vi "Protocol.Initialize.vi"(8 "error in (no error)":errorcluster, 10 "Parameters in":T21={"Name"="", "XNET.Settings"={"Database"="", "Cluster"="", "Port"="", "Baud rate [Bd]"=0, "Termination"=0, "Incoming Decimation"=0, "Outgoing Decimation"=1}, "Monitor.Network"={"Address"=0, "Name"=0, "Include DA"=FALSE}, "Data"=[], "DTCs"=[], "Sim.Nodes.LUT"=variant, "Data.LUT"=variant, "PCL"=0} {"Monitor.Network"."Name" format="%.0x"; "DTCs"."Data"."DM1.Ref"."Data Reference" format="%.0x"; "DTCs"."Data"."DM1.Enable.Ref"."Data Reference" format="%.0x"; "DTCs"."Data"."DM2.Ref"."Data Reference" format="%.0x"; "DTCs"."Data"."DM2.Enable.Ref"."Data Reference" format="%.0x"; "Data"."Trigger.Refs"."Data Reference" format="%.0x"; "Data"."Disable.Refs"."Data Reference" format="%.0x"; "Data"."Timing.Refs"."Data Reference" format="%.0x"; "Data"."Network"."Name" format="%.0x"; "Data"."Incoming.Refs"."Data Reference" format="%.0x"; "Data"."Outgoing.Refs"."Data Reference" format="%.0x"; "XNET.Settings"."Termination" items=["Off", "On"]}, 11 "Process":refnum<class "Process.lvclass">) -> (0 "error out":errorcluster, 2 "Notification":bool, 3 "Protocol State Variables":T1 {"Stream Refs"."Port Settings"."FD ISO Mode" items=["ISO", "Non ISO", "ISO Legacy"]; "Stream Refs"."Port Settings"."Termination" items=["Off", "On"]; "Stream Refs"."Port Settings"."Mode" items=["CAN 2.0", "CAN FD", "CAN FD+BRS"]})   [LabVIEW 2019, in "J1939 Addon Engine.lvlib"]
uses:
  J1939 Addon Engine.lvlib
  Support Libraries/J1939 Utilities/Types/CAN Outgoing Message Cluster.ctl
  Support Libraries/J1939 Utilities/J1939 Utilities.lvlib
  Types/Protocol.Refs.ctl
  Types/Protocol.Configuration.ctl
  Types/Protocol.XNET Settings.ctl
  Types/Protocol.Address Table Reference.ctl
  Types/Protocol.RQST Lookup Table Reference.ctl
  <vilib>/NI/NI VeriStand Addon Network Comm/Engine/VeriStand Comm.lvclass
  <vilib>/NI/NIVS Inline Async API/_VS Inline Async API/Process/Process.lvclass
  <vilib>/NI/NIVS Inline Async API/_Data Access Engine/Access Type Classes/Write/Write.lvclass
  <vilib>/NI/NIVS Inline Async API/_Data Access Engine/Data Access Engine/Types/Write.DVR.ctl
  <vilib>/NI/NIVS Inline Async API/_Data Access Engine/Data Access Engine/Data Access Engine.lvclass
  <vilib>/NI/NIVS Inline Async API/_Data Access Engine/Access Type Classes/Read/Read.lvclass
  <vilib>/NI/NIVS Inline Async API/_Data Access Engine/Data Access Engine/Types/Read.DVR.ctl
  Addon Shared/SubVIs/Constants.vi
  Addon Shared/J1939 Addon Shared.lvlib
  SubModules/Frame-Protection-Support/Source/Engine/Types/RT Frame Settings.ctl
  SubModules/Frame-Protection-Support/Source/Engine/Protection and Counter Support Engine.lvlib
  Types/CounterAndProtectionFrames.ctl
  <vilib>/NI/NIVS Inline Async API/_Data Access Engine/Data Access Engine/Methods/Write.Lookup.vi
  <vilib>/NI/NIVS Inline Async API/_Data Access Engine/Data Access Engine/Methods/Read.Lookup.vi
  SubModules/Frame-Protection-Support/Source/Shared/Types/Exported Event Trigger Type.ctl
  SubModules/Frame-Protection-Support/Source/Shared/Protection and Counter Support Shared.lvlib
  SubModules/Frame-Protection-Support/Source/Shared/Types/Exported Counter Settings.ctl
  SubModules/Frame-Protection-Support/Source/Shared/Types/XNET Signal Configuration.ctl
  SubModules/Frame-Protection-Support/Source/Shared/Types/Protection Type.ctl
  SubModules/Frame-Protection-Support/Source/Engine/Types/RT Protection Configuration.ctl
  SubModules/Frame-Protection-Support/Source/Shared/Types/Exported Frame Type.ctl
  SubModules/CAN-Streaming-Support/Source/Addon/Addon Shared/Types/Type Filter.ctl
  SubModules/CAN-Streaming-Support/Source/Addon/Addon Shared/CAN Stream Support Shared.lvlib
  SubModules/CAN-Streaming-Support/Source/Addon/Addon Shared/Types/Direction Filter.ctl
  SubModules/CAN-Streaming-Support/Source/Addon/Addon Shared/Types/Filter Parameters.ctl
  SubModules/CAN-Streaming-Support/Source/Addon/Addon Engine/Types/Engine Stream Refs.ctl
  SubModules/CAN-Streaming-Support/Source/Addon/Addon Engine/CAN Stream Support Engine.lvlib
  SubModules/CAN-Streaming-Support/Source/Addon/Addon Engine/Types/Engine Stream Port Settings.ctl
  <vilib>/NI VeriStand/Custom Device API/Data Reference.ctl
  <vilib>/NI VeriStand/Custom Device API/Custom Device API.lvlib
  Addon Shared/Types/XNET Settings.ctl
  <vilib>/NI VeriStand/Custom Device API/Block Data Reference.ctl
  Types/Protocol.App Settings.ctl
  Addon Shared/Types/Compiled Simulated Settings.ctl
  Types/Engine.DTC FIFOs.ctl
  Types/Engine.DTC Settings.ctl
  Types/Protocol.XNET Refs.ctl
  Addon Shared/Types/Monitor Settings.ctl
  Types/Main.Outgoing.Frame.Settings.ctl
  Addon Shared/Types/Outgoing Event Trigger Types.ctl
  SubModules/Frame-Protection-Support/Source/Shared/Types/Exported Frame Settings.ctl
  SubModules/Frame-Protection-Support/Source/Shared/Types/Exported Protection Settings.ctl
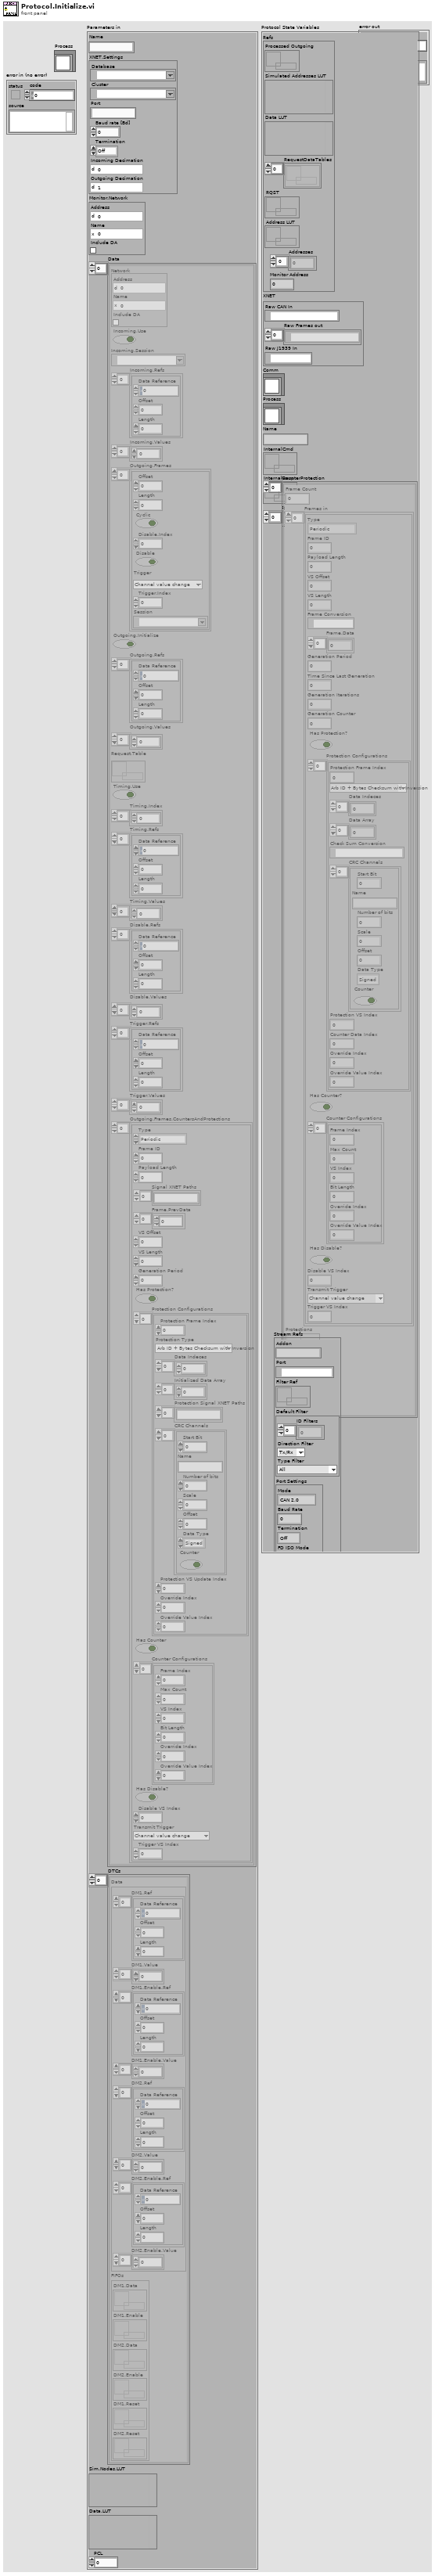
[diagram p1: front panel]
types:
  T1 = typedef "J1939 Addon Engine.lvlib/Protocol.Configuration.ctl" = cluster{"Refs":T2, "XNET":T5, "Comm":refnum<class "VeriStand Comm.lvclass">, "Process":refnum<class "Process.lvclass">, "Name":string, "InternalCmd":T6, "InternalResp":T7, "Resp.Data":dbl[], "CounterProtection":T8[], "Stream Refs":T16}
  T2 = typedef "J1939 Addon Engine.lvlib/Protocol.Refs.ctl" = cluster{"Processed Outgoing":refnum<queue>, "Simulated Addresses LUT":variant, "Data LUT":variant, "RequestDataTables":refnum<k33>[], "RQST":T3, "Address LUT":T4, "Addresses":u8[], "Monitor Address":u8}
  T3 = typedef "J1939 Addon Engine.lvlib/Protocol.RQST Lookup Table Reference.ctl" = refnum<data-value>
  T4 = typedef "J1939 Addon Engine.lvlib/Protocol.Address Table Reference.ctl" = refnum<data-value>
  T5 = typedef "J1939 Addon Engine.lvlib/Protocol.XNET Settings.ctl" = cluster{"Raw CAN In":refnum<k21>, "Raw Frames out":refnum<k21>[], "Raw J1939 In":refnum<k21>}
  T6 = typedef "Data Access Engine.lvlib/Data Access Engine.lvclass/Read.DVR.ctl" = refnum<data-value>
  T7 = typedef "Data Access Engine.lvlib/Data Access Engine.lvclass/Write.DVR.ctl" = refnum<data-value>
  T8 = typedef "J1939 Addon Engine.lvlib/CounterAndProtectionFrames.ctl" = cluster{"Frame Count":i32, "Frames in":T9[], "Protections":T7, "Signals":T6, "Overrides":T6}
  T9 = typedef "Protection and Counter Support Engine.lvlib/RT Frame Settings.ctl" = cluster{"Type":T10, "Frame ID":u32, "Payload Length":u32, "VS Offset":i32, "VS Length":i32, "Frame Conversion":refnum<k21>, "Frame.Data":dbl[], "Generation Period":u32, "Time Since Last Generation":u32, "Generation Iterations":u32, "Generation Counter":u32, "Has Protection?":bool, "Protection Configurations":T11[], "Has Counter?":bool, "Counter Configurations":T14[], "Has Disable?":bool, "Disable VS Index":i32, "Transmit Trigger":T15, "Trigger VS Index":i32}
  T10 = typedef "Protection and Counter Support Shared.lvlib/Exported Frame Type.ctl" = enum16{"Periodic", "Event", "Periodic/Event"}
  T11 = typedef "Protection and Counter Support Engine.lvlib/RT Protection Configuration.ctl" = cluster{"Protection Frame Index":i32, "Protection Type":T12, "Data Indeces":i32[], "Data Array":dbl[], "Check Sum Conversion":refnum<k21>, "CRC Channels":T13[], "Protection VS Index":i32, "Counter Data Index":i32, "Override Index":i32, "Override Value Index":i32}
  T12 = typedef "Protection and Counter Support Shared.lvlib/Protection Type.ctl" = enum16{"Arb ID + Bytes Checksum with Inversion", "Arb ID + Bytes CRC with Inversion", "Reversed Raw Signal Checksum with Inversion", "Concatenated Two's Compliment"}
  T13 = typedef "Protection and Counter Support Shared.lvlib/XNET Signal Configuration.ctl" = cluster{"Start Bit":i32, "Name":string, "Number of bits":i32, "Scale":dbl, "Offset":dbl, "Data Type":u32, "Counter":bool}
  T14 = typedef "Protection and Counter Support Shared.lvlib/Exported Counter Settings.ctl" = cluster{"Frame Index":i32, "Max Count":dbl, "VS Index":i32, "Bit Length":i64, "Override Index":i32, "Override Value Index":i32}
  T15 = typedef "Protection and Counter Support Shared.lvlib/Exported Event Trigger Type.ctl" = enum16{"Channel value change", "Trigger channel (not zero)", "Channel value change or trigger channel (not zero)", "Trigger channel (any value change)", "Channel value change or trigger channel (any value change)"}
  T16 = typedef "CAN Stream Support Engine.lvlib/Engine Stream Refs.ctl" = cluster{"Addon":string, "Port":refnum<k21>, "Filter Ref":refnum<data-value>, "Default Filter":T17, "Port Settings":T20}
  T17 = typedef "CAN Stream Support Shared.lvlib/Filter Parameters.ctl" = cluster{"ID Filters":u32[], "Direction Filter":T18, "Type Filter":T19}
  T18 = typedef "CAN Stream Support Shared.lvlib/Direction Filter.ctl" = enum16{"Tx/Rx", "Rx", "Tx"}
  T19 = typedef "CAN Stream Support Shared.lvlib/Type Filter.ctl" = enum16{"All", "CAN Data", "CAN Remote", "CAN Bus Error", "CAN 2.0 Data", "CAN FD Data", "CAN FD+BRS Data", "J1939 Data", "Delay", "Log Trigger", "Start Trigger"}
  T20 = typedef "CAN Stream Support Engine.lvlib/Engine Stream Port Settings.ctl" = cluster{"Mode":u32, "Baud Rate":u64, "Termination":u32, "FD ISO Mode":u32, "FD Baud Rate":u64}
  T21 = typedef "J1939 Addon Engine.lvlib/Protocol.App Settings.ctl" = cluster{"Name":string, "XNET.Settings":T22, "Monitor.Network":T23, "Data":T24[], "DTCs":T31[], "Sim.Nodes.LUT":variant, "Data.LUT":variant, "PCL":u32}
  T22 = typedef "J1939 Addon Shared.lvlib/XNET Settings.ctl" = cluster{"Database":refnum<k21>, "Cluster":refnum<k21>, "Port":string, "Baud rate [Bd]":u32, "Termination":u32, "Incoming Decimation":u32, "Outgoing Decimation":u32}
  T23 = typedef "J1939 Addon Shared.lvlib/Monitor Settings.ctl" = cluster{"Address":u8, "Name":u64, "Include DA":bool}
  T24 = typedef "J1939 Addon Engine.lvlib/Protocol.XNET Refs.ctl" = cluster{"Network":T23, "Incoming.Use":bool, "Incoming.Session":refnum<k21>, "Incoming.Refs":T25[], "Incoming.Values":dbl[], "Outgoing.Frames":T27[], "Outgoing.Initialize":bool, "Outgoing.Refs":T25[], "Outgoing.Values":dbl[], "Request.Table":refnum<k33>, "Timing.Use":bool, "Timing.Index":i32[], "Timing.Refs":T25[], "Timing.Values":dbl[], "Disable.Refs":T25[], "Disable.Values":dbl[], "Trigger.Refs":T25[], "Trigger.Values":dbl[], "Outgoing.Frames.CountersAndProtections":T29[]}
  T25 = typedef "Custom Device API.lvlib/Block Data Reference.ctl" = cluster{"Data Reference":T26, "Offset":u64, "Length":u64}
  T26 = typedef "Custom Device API.lvlib/Data Reference.ctl" = i32
  T27 = typedef "J1939 Addon Engine.lvlib/Main.Outgoing.Frame.Settings.ctl" = cluster{"Offset":u32, "Length":u32, "Cyclic":bool, "Disable.Index":i32, "Disable":bool, "Trigger":T28, "Trigger.Index":i32, "Session":refnum<k21>}
  T28 = typedef "J1939 Addon Shared.lvlib/Outgoing Event Trigger Types.ctl" = enum16{"Channel value change", "Trigger channel (not zero)", "Channel value change or trigger channel (not zero)", "Trigger channel (any value change)", "Channel value change or trigger channel (any value change)"}
  T29 = typedef "Protection and Counter Support Shared.lvlib/Exported Frame Settings.ctl" = cluster{"Type":T10, "Frame ID":u32, "Payload Length":u32, "Signal XNET Paths":string[], "Frame.PrevData":dbl[], "VS Offset":i32, "VS Length":i32, "Generation Period":u32, "Has Protection?":bool, "Protection Configurations":T30[], "Has Counter":bool, "Counter Configurations":T14[], "Has Disable?":bool, "Disable VS Index":i32, "Transmit Trigger":T15, "Trigger VS Index":i32}
  T30 = typedef "Protection and Counter Support Shared.lvlib/Exported Protection Settings.ctl" = cluster{"Protection Frame Index":i32, "Protection Type":T12, "Data Indeces":i32[], "Initialized Data Array":dbl[], "Protection Signal XNET Paths":string[], "CRC Channels":T13[], "Protection VS Update Index":i32, "Override Index":i32, "Override Value Index":i32}
  T31 = typedef "J1939 Addon Engine.lvlib/Engine.DTC Settings.ctl" = cluster{"Data":T32, "FIFOs":T33}
  T32 = typedef "J1939 Addon Shared.lvlib/Compiled Simulated Settings.ctl" = cluster{"DM1.Ref":T25[], "DM1.Value":dbl[], "DM1.Enable.Ref":T25[], "DM1.Enable.Value":dbl[], "DM2.Ref":T25[], "DM2.Value":dbl[], "DM2.Enable.Ref":T25[], "DM2.Enable.Value":dbl[]}
  T33 = typedef "J1939 Addon Engine.lvlib/Engine.DTC FIFOs.ctl" = cluster{"DM1.Data":refnum<k33>, "DM1.Enable":refnum<k33>, "DM2.Data":refnum<k33>, "DM2.Enable":refnum<k33>, "DM1.Reset":refnum<k33>, "DM2.Reset":refnum<k33>}
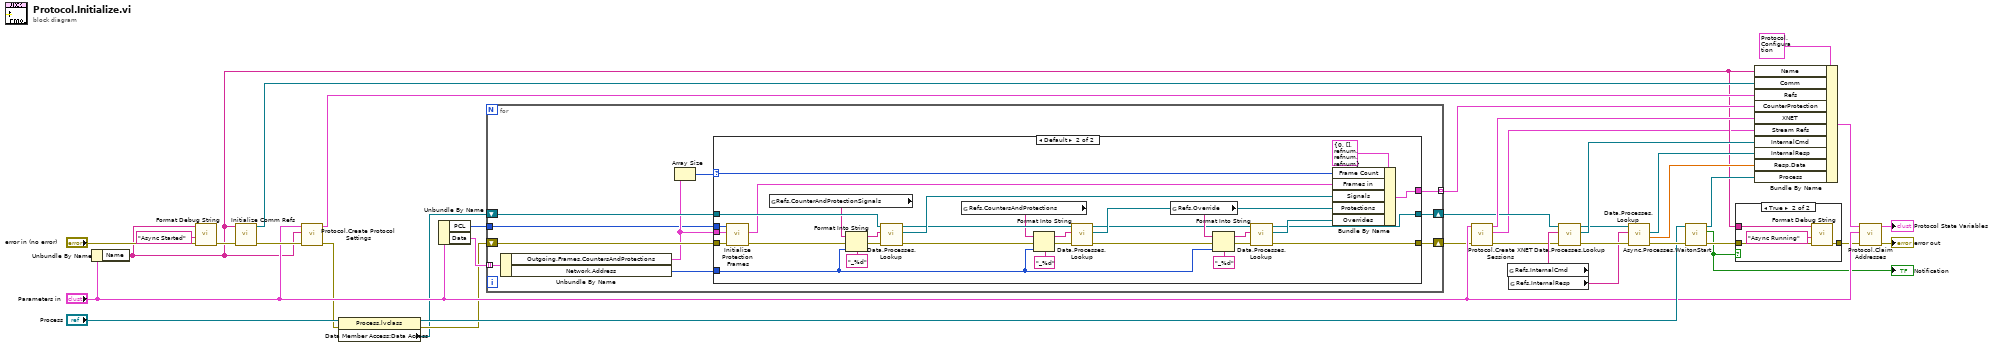
[diagram p0: block diagram]
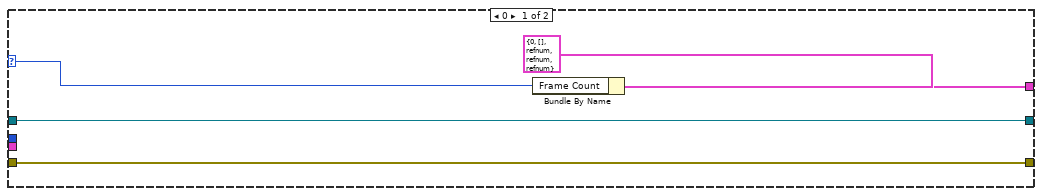
[diagram p3: hidden frame]
diagram:
  n1 = Unbundle By Name("Parameters in") -> ("Name"=w2:string)
  n2 = call "Format Debug String.vi"("error in (no error)"="error in (no error)", "State"="Async Started", "Name"=w2) -> ("error out"=w6:errorcluster)  [unwired: 8 in]
  n3 = call <vilib>:"Initialize Comm Refs.vi"("error in (no error)"=w6, "Name"=w2) -> ("error out"=w34:errorcluster, "Comm.lvclass"=w33:refnum<class "VeriStand Comm.lvclass">)  [unwired: 8 in]
  n4 = call "Protocol.Create Protocol Settings.vi"("error in (no error)"=w34, "Name in"=w2, "Parameters in"="Parameters in") -> ("error out"=w15:errorcluster, "Protocol Refs"=w9:T2)  [unwired: 7 in]
  n5 = property class="Process.lvclass"(reference="Process", error in=w15) -> (reference out=w23:refnum<class "Process.lvclass">, error out=w14:errorcluster, "Data Member Access:Data Access"=w12:refnum<class "Data Access Engine.lvclass">)
  n6 = Unbundle By Name("Parameters in") -> ("PCL"=w10:u32, "Data"=w17:T24[])
  n7 = for {
    shift-right: [w46] -> w18
    shift-left: w14 -> [w40]
    tunnel: w17 -> [w47] mode=indexing
    tunnel: [w45] -> w16 mode=indexing
    shift-right: [w43] -> w11
    shift-left: w12 -> [w44]
    tunnel: w10 -> [w38]
    n8 = Unbundle By Name(w47) -> ("Outgoing.Frames.CountersAndProtections"=w39:T29[], "Network.Address"=w42:u8)
    n9 = Array Size(array=w39) -> (size(s)=w41:i32)
    n10 = case shown="Default" w41 {
      selector: w41 -> [w48 w68]
      tunnel: [w52 w57] -> w46
      tunnel: [w50 w82] -> w45
      tunnel: w44 -> [w49 w79]
      tunnel: [w49 w53] -> w43
      tunnel: w40 -> [w52 w67]
      tunnel: w39 -> [_ w65]
      tunnel: w42 -> [_ w56]
      tunnel: w38 -> [_ w66]
      frame 0 {
        n11 = Bundle By Name(cluster=T8 {"Frame Count"=0, "Frames in"=[], "Protections"=refnum, "Signals"=refnum, "Overrides"=refnum}, "Frame Count"=w48) -> (w50:T8)
      }
      frame Default {
        n12 = call "Initialize Protection Frames.vi"("error in (no error)"=w67, "Frames"=w65, "PCL (usec)"=w66) -> ("error out"=w63:errorcluster, "RT Frames"=w64:T9[])  [unwired: 7 in]
        n13 = global read "Constants.vi" "Refs.CounterAndProtectionSignals"() -> (w73:string)
        n14 = Format Into String(format string="_%d", initial string=w73, error in=w63, w56) -> (resulting string=w71:string, error out=w77:errorcluster)
        n15 = call-poly <vilib>:"Data.Processes.Lookup.vi"("error in (no error)"=w77, "Name"=w71, "Data Access API in"=w79) -> ("error out"=w76:errorcluster, "Ref"=w80:T6, "Data Access API out"=w78:refnum<class "Data Access Engine.lvclass">)  [unwired: 5 in, 1 out]
        n16 = global read "Constants.vi" "Refs.CountersAndProtections"() -> (w70:string)
        n17 = Format Into String(format string="_%d", initial string=w70, error in=w76, w56) -> (resulting string=w74:string, error out=w75:errorcluster)
        n18 = call-poly <vilib>:"Data.Processes.Lookup.vi"("error in (no error)"=w75, "Name"=w74, "Data Access API in"=w78) -> ("error out"=w58:errorcluster, "Ref"=w81:T7, "Data Access API out"=w54:refnum<class "Data Access Engine.lvclass">)  [unwired: 5 in, 1 out]
        n19 = global read "Constants.vi" "Refs.Override"() -> (w61:string)
        n20 = Format Into String(format string="_%d", initial string=w61, error in=w58, w56) -> (resulting string=w60:string, error out=w59:errorcluster)
        n21 = call-poly <vilib>:"Data.Processes.Lookup.vi"("error in (no error)"=w59, "Name"=w60, "Data Access API in"=w54) -> ("error out"=w57:errorcluster, "Ref"=w55:T6, "Data Access API out"=w53:refnum<class "Data Access Engine.lvclass">)  [unwired: 5 in, 1 out]
        n22 = Bundle By Name(cluster=T8 {"Frame Count"=0, "Frames in"=[], "Protections"=refnum, "Signals"=refnum, "Overrides"=refnum}, "Frame Count"=w68, "Frames in"=w64, "Signals"=w80, "Protections"=w81, "Overrides"=w55) -> (w82:T8)
      }
    }
  }
  n23 = call "Protocol.Create XNET Sessions.vi"("error in (no error)"=w18, "Parameters in"="Parameters in") -> ("error out"=w13:errorcluster, "Stream Refs"=w1:T16, "XNET"=w36:T5)  [unwired: 7 in]
  n24 = global read "Constants.vi" "Refs.InternalCmd"() -> (w21:string)
  n25 = global read "Constants.vi" "Refs.InternalResp"() -> (w22:string)
  n26 = call-poly <vilib>:"Data.Processes.Lookup.vi"("error in (no error)"=w13, "Name"=w21, "Data Access API in"=w11) -> ("error out"=w26:errorcluster, "Ref"=w29:T6, "Data Access API out"=w25:refnum<class "Data Access Engine.lvclass">)  [unwired: 5 in, 1 out]
  n27 = call-poly <vilib>:"Data.Processes.Lookup.vi"("error in (no error)"=w26, "Name"=w22, "Data Access API in"=w25) -> ("error out"=w27:errorcluster, "Initial Values"=w28:dbl[], "Ref"=w30:T7)  [unwired: 5 in, 1 out]
  n28 = call <vilib>:"Async.Processes.WaitonStart.vi"("error in (no error)"=w27, "Process"=w23) -> ("error out"=w5:errorcluster, "Execute"=w3:bool, "Process out"=w32:refnum<class "Process.lvclass">)  [unwired: 7 in]
  "Notification" <- w3
  n29 = case shown="True" w3 {
    tunnel: w5 -> [w84 w87]
    tunnel: [w84 w86] -> w4
    tunnel: w2 -> [_ w85]
    frame False {
    }
    frame True {
      n30 = call "Format Debug String.vi"("error in (no error)"=w87, "State"="Async Running", "Name"=w85) -> ("error out"=w86:errorcluster)  [unwired: 8 in]
    }
  }
  n31 = Bundle By Name(cluster=T1 {"Refs"={"Processed Outgoing"=refnum, "Simulated Addresses LUT"=variant, "Data LUT"=variant, "RequestDataTables"=[], "RQST"=refnum, "Address LUT"=refnum, "Addresses"=[], "Monitor Address"=0}, "XNET"={"Raw CAN In"="", "Raw Frames out"=[], "Raw J1939 In"=""}, "Comm"=refnum, "Process"=refnum, "Name"="", "InternalCmd"=refnum, "InternalResp"=refnum, "Resp.Data"=[], "CounterProtection"=[], "Stream Refs"={"Addon"="", "Port"="", "Filter Ref"=refnum, "Default Filter"={"ID Filters"=[], "Direction Filter"=enum."Tx/Rx", "Type Filter"=enum."All"}, "Port Settings"={"Mode"=0, "Baud Rate"=0, "Termination"=0, "FD ISO Mode"=0, "FD Baud Rate"=0}}} ("output cluster"), "Name"=w2, "Comm"=w33, "Refs"=w9, "CounterProtection"=w16, "XNET"=w36, "Stream Refs"=w1, "InternalCmd"=w29, "InternalResp"=w30, "Resp.Data"=w28, "Process"=w32) -> (w20:T1)
  n32 = call "Protocol.Claim Addresses.vi"("error in"=w4, "Parameters in"="Parameters in", "J1939 Main Configuration"=w20) -> ("error out"=→"error out":errorcluster, "output cluster"=→"Protocol State Variables":T1)  [unwired: 7 in]
